vi "RLS_identificacion.vi"() -> ()   [LabVIEW 2022 SP3]
uses:
  <vilib>/Utility/NIReport.llb/Report Type.ctl
  <vilib>/imath/engines/lvmath2/RunTimeEngine/NodeEndStatement/NIMS_NodeEndStatement_Output.vi
  <instcachedir>/0/NIMS_NodeEndStatement_Output_53EC0D466D134D7ABD903AC30B43404B.lvgen/NIMS_NodeEndStatement_Output_53EC0D466D134D7ABD903AC30B43404B_001.vi
  <vilib>/imath/engines/lvmath2/RunTimeEngine/ErrorHandling/NIMS_Finalize Error.vi
  <vilib>/imath/engines/lvmath2/RunTimeEngine/Managers/WorkSpace/UID Generator.vi
  <vilib>/imath/engines/lvmath2/RunTimeEngine/RunTimeType/NIMS_RunTimeType_From StrictType (excl LVString).vi
  <instcachedir>/0/NIMS_RunTimeType_From StrictType (excl LVString)_70DEE8F51B6B495C85F505DE4E7061F1.lvgen/NIMS_RunTimeType_From StrictType (excl LVString)_70DEE8F51B6B495C85F505DE4E7061F1_000.vi
  <vilib>/imath/engines/lvmath2/RunTimeEngine/LocalVariableDefStatement/MC_LocalVariableDefStatement_Display.vi
  <vilib>/imath/engines/lvmath2/RunTimeEngine/ArithmeticOperatorToken/NIMS_ArithmeticOperator_multmx(RV,M).vi
  <instcachedir>/0/NIMS_ArithmeticOperator_multmx(RV,M)_0C5EC56C64A44F5D9A149E640905A95E.lvgen/NIMS_ArithmeticOperator_multmx(RV,M)_0C5EC56C64A44F5D9A149E640905A95E_001.vi
  <vilib>/imath/engines/lvmath2/RunTimeEngine/ArithmeticOperatorToken/NIMS_ArithmeticOperator_multmx(M,CV).vi
  <instcachedir>/0/NIMS_ArithmeticOperator_multmx(M,CV)_F5DBFFF0126A4383B39F7B34D5ABA6C8.lvgen/NIMS_ArithmeticOperator_multmx(M,CV)_F5DBFFF0126A4383B39F7B34D5ABA6C8_000.vi
  <vilib>/imath/engines/lvmath2/RunTimeEngine/ArithmeticOperatorToken/NIMS_ArithmeticOperator_rightdivmx.vi
  <instcachedir>/0/NIMS_ArithmeticOperator_rightdivmx_6089A681D87747958E3B9B6C89182D1F.lvgen/NIMS_ArithmeticOperator_rightdivmx_6089A681D87747958E3B9B6C89182D1F_000.vi
  <vilib>/imath/engines/lvmath2/RunTimeEngine/ErrorHandling/NIMS_Create Error From Enums.vi
  <vilib>/imathl/engines/lvmath/Functions/Error Handling/Create Error.vi
  <vilib>/imath/engines/lvmath2/RunTimeEngine/ArithmeticOperatorToken/NIMS_ArithmeticOperator_multmx.vi
  <instcachedir>/0/NIMS_ArithmeticOperator_multmx_BDE1B5075EB4429787EED704427CBD98.lvgen/NIMS_ArithmeticOperator_multmx_BDE1B5075EB4429787EED704427CBD98_004.vi
  <vilib>/imath/engines/lvmath2/RunTimeEngine/ArithmeticOperatorToken/NIMS_ArithmeticOperator_plus.vi
  <instcachedir>/0/NIMS_ArithmeticOperator_plus_3E2F46F6B6A2434E909AF418D4802C21.lvgen/NIMS_ArithmeticOperator_plus_3E2F46F6B6A2434E909AF418D4802C21_003.vi
  <vilib>/imath/engines/lvmath2/RunTimeEngine/ArithmeticOperatorToken/NIMS_ArithmeticOperator_minus.vi
  <instcachedir>/0/NIMS_ArithmeticOperator_minus_22EE3FD1C8824638A4ED1C446A3DB56D.lvgen/NIMS_ArithmeticOperator_minus_22EE3FD1C8824638A4ED1C446A3DB56D_009.vi
  <vilib>/imath/engines/lvmath2/RunTimeEngine/IndexRead/NIMS M(S).vi
  <instcachedir>/0/NIMS M(S)_B826C018497E4940AE96BD27B540B6FB.lvgen/NIMS M(S)_B826C018497E4940AE96BD27B540B6FB_000.vi
  <vilib>/imath/engines/lvmath2/RunTimeEngine/Managers/SymbolTable/Clear UID.vi
  <instcachedir>/0/NIMS_NodeEndStatement_Output_53EC0D466D134D7ABD903AC30B43404B.lvgen/NIMS_NodeEndStatement_Output_53EC0D466D134D7ABD903AC30B43404B_002.vi
  <vilib>/addons/_office/excel.llb/Excel Easy Table (num).vi
  <vilib>/Utility/NIReport.llb/NI_report.lvclass
  <vilib>/Utility/NIReport.llb/NI_ReportGenerationCore.lvlib
  <vilib>/Utility/NIReport.llb/Excel/NI_Excel.lvclass
  <vilib>/addons/_office/NI_ReportGenerationToolkit.lvlib
  <vilib>/imath/engines/lvmath2/RunTimeEngine/Managers/SymbolTable/NIMS_WorkSpace.lvlib
panel:
  in  "template (empty)":path
  in  "stop":bool
  in  "u(k)":dbl
  in  "Pertubación":bool
  in  "Tiempo de  ejecucion":u32
  out "ARX orden 2":cluster{"set-point ":dbl, dbl, dbl, dbl}(graph)
  out "tetak2":dbl[][](array[numeric])
  out "ARX orden 1":cluster{"set-point ":dbl, dbl, dbl, dbl}(graph)
  out "tetak":dbl[][](array[numeric])
  out "a11":dbl
  out "a1":dbl=-0.8261
  out "a2":dbl
  out "b1":dbl=0.008316
  out "b2":dbl=0.1498
  out "b11":dbl
  out "a12":dbl
  out "a22":dbl
  out "b12":dbl
  out "?":dbl
  # "Vector de parametros\nestimados"
  # "Vector de parametros\nestimados"
  # "Z+"
  # "Gp(Z) ="
  # "Gp(Z) ="
  # "Z +"
  # "Z^2 +"
  # "Z+"
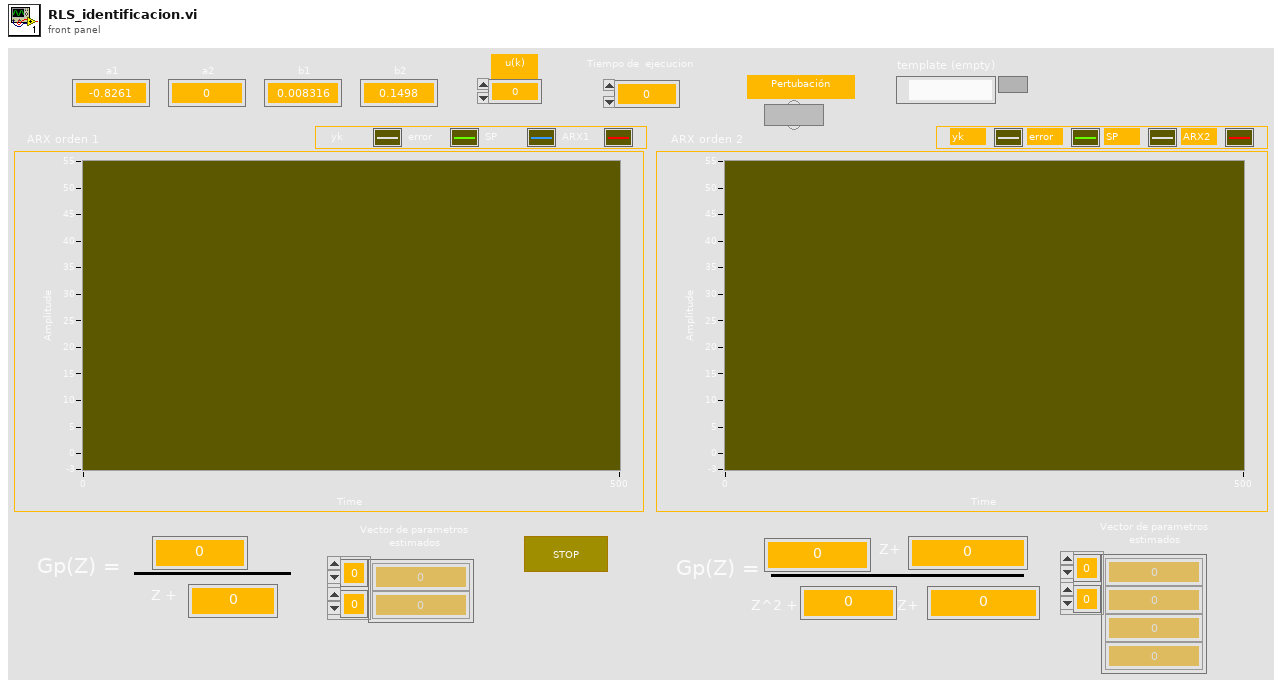
[diagram p1: front panel]
types:
  T1 = typedef "NI_ReportGenerationCore.lvlib/Report Type.ctl" = enum16{"HTML", "Word", "Excel"}
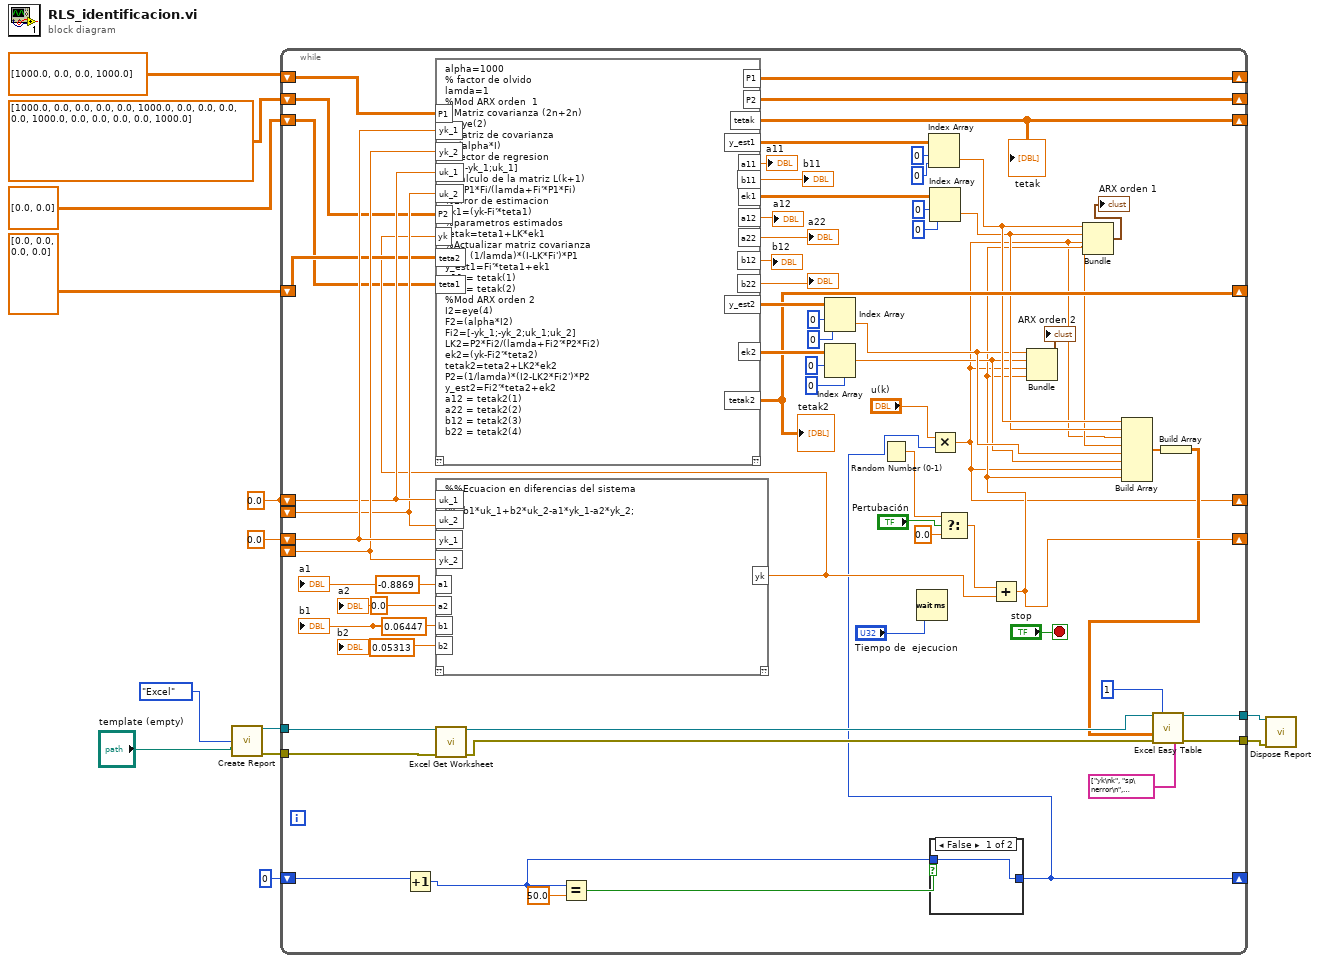
[diagram p0: block diagram]
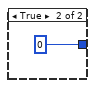
[diagram p2: hidden frame]
diagram:
  w9 = 0.0 ("set-point")
  w8 = 0.0 ("set-point")
  n1 = call <vilib>:"Create Report.vi"("report type"=Report_Type."Excel", "template (empty)"="template (empty)") -> ("report out"=w5:refnum<class "NI_report.lvclass">, "error out"=w4:errorcluster)  [unwired: 12 in]
  n2 = while {
    shift-right: [w29] -> _
    shift-left: w8 -> [w77]
    shift-left: w8 -> [w76]
    shift-right: [w19] -> _
    shift-left: w9 -> [w75]
    shift-left: w9 -> [w74]
    shift-right: [w59] -> _
    shift-left: dbl[][] [[0.0], [0.0], [0.0], [0.0]] ("tetak2") -> [w73]
    shift-right: [w58] -> _
    shift-left: dbl[][] [[1000.0, 0.0], [0.0, 1000.0]] ("P1") -> [w56]
    shift-right: [w57] -> _
    shift-left: dbl[][] [[1000.0, 0.0, 0.0, 0.0], [0.0, 1000.0, 0.0, 0.0], [0.0, 0.0, 1000.0, 0.0], [0.0, 0.0, 0.0, 1000.0]] ("P") -> [w55]
    shift-right: [w54] -> _
    shift-left: dbl[][] [[0.0], [0.0]] ("tetak") -> [w53]
    tunnel: w5 -> [w35]
    tunnel: w4 -> [w34]
    tunnel: [w22] -> w3
    tunnel: [w21] -> w2
    shift-right: [w14] -> _
    shift-left: 0 -> [w18]
    stop <- "stop" stop-if-true
    w41 = 0.05313 ("b2")
    w42 = 0.06447 ("b1")
    w43 = 0.0 ("a2")
    w44 = -0.8869 ("a1")
    n3 = Increment(x=w18) -> (x+1=w15:i32)
    n4 = mathscript code="%%Ecuacion en diferencias del sistema\n\nyk=b1*uk_1+b2*uk_2-a1*yk_1-a2*yk_2;"("uk_1"=w75, "uk_2"=w74, "yk_1"=w77, "yk_2"=w76, "a1"=w44, "a2"=w43, "b1"=w42, "b2"=w41) -> ("yk"=w62:dbl)  [unwired: 1 in, 1 out]
    n5 = mathscript code="alpha=1000\n% factor de olvido \nlamda=1\n%Mod ARX orden  1\n%Matriz covarianza (2n+2n)\nI=eye(2)\n%Matriz de covarianza \nF=(alpha*I)\n%Vector de regresion\nFi=[-yk_1;uk_1]\n%Calculo de la matriz L(k+1)\nLK=P1*Fi/(lamda+Fi'*P1*Fi)\n%Error de estimacion \nek1=(yk-Fi'*teta1)\n%parametros estimados \ntetak=teta1+LK*ek1\n%Actualizar matriz covarianza \nP1 = (1/lamda)*(I-LK*Fi')*P1\ny_est1=Fi'*teta1+ek1\na11 = tetak(1)\nb11 = tetak(2)\n%Mod ARX orden 2\nI2=eye(4)\nF2=(alpha*I2)\nFi2=[-yk_1;-yk_2;uk_1;uk_2]\nLK2=P2*Fi2/(lamda+Fi2'*P2*Fi2)\nek2=(yk-Fi2'*teta2)\ntetak2=teta2+LK2*ek2\nP2=(1/lamda)*(I2-LK2*Fi2')*P2\ny_est2=Fi2'*teta2+ek2\na12 = tetak2(1)\na22 = tetak2(2)\nb12 = tetak2(3)\nb22 = tetak2(4)"("yk_1"=w77, "yk_2"=w76, "uk_1"=w75, "uk_2"=w74, "P2"=w55, "yk"=w62, "teta2"=w73, "teta1"=w53, "P1"=w56) -> ("tetak2"=w59:dbl[][], "ek2"=w66:dbl[][], "y_est2"=w60:dbl[][], "P1"=w58:dbl[][], "P2"=w57:dbl[][], "tetak"=w54:dbl[][], "ek1"=w49:dbl[][], "y_est1"=w51:dbl[][], "a11"=→"a11":dbl, "b11"=→"b11":dbl, "a12"=→"a12":dbl, "a22"=→"a22":dbl, "b12"=→"b12":dbl, "b22"=→"?":dbl)  [unwired: 1 in, 1 out]
    "tetak2" <- w59
    "tetak" <- w54
    n6 = call <vilib>:"Excel Get Worksheet.vi"("report in"=w35, "error in (no error)"=w34) -> ("report out"=w25:refnum<class "NI_report.lvclass">, "error out"=w24:errorcluster)  [unwired: 12 in]
    n7 = Equal?(x=w15, y=50.0) -> (x = y?=w16:bool)
    n8 = Index Array(array=w60, index (row)=0 ("disabled index (row)"), index (col)=0 ("disabled index (col)")) -> (element=w31:dbl)
    n9 = Index Array(array=w66, index (row)=0, index (col)=0 ("disabled index (col)")) -> (element=w30:dbl)
    n10 = Random Number (0-1)() -> (number: 0 to 1=w67:dbl)
    n11 = Wait (ms)(milliseconds to wait="Tiempo de  ejecucion") -> ()  [unwired: 1 out]
    n12 = Index Array(array=w51, index (row)=0 ("disabled index (row)"), index (col)=0 ("disabled index (col)")) -> (element=w33:dbl)
    n13 = Index Array(array=w49, index (row)=0 ("disabled index (row)"), index (col)=0 ("disabled index (col)")) -> (element=w32:dbl)
    n14 = case shown="False" w16 {
      tunnel: [w79 0] -> w14
      tunnel: w15 -> [w79 _]
      frame False {
      }
      frame True {
      }
    }
    n15 = Multiply(x="u(k)", y=w14) -> (x*y=w19:dbl)
    n16 = Select(t=w67, s="Pertubación", f=0.0) -> (s? t:f=w68:dbl)
    n17 = Add(x=w68, y=w62) -> (x+y=w29:dbl)
    n18 = Bundle(w31, w30, w19, w29) -> (→"ARX orden 2":cluster{dbl, dbl, dbl, dbl})  [unwired: 1 in]
    n19 = Bundle(w33, w32, w19, w29) -> (→"ARX orden 1":cluster{dbl, dbl, dbl, dbl})  [unwired: 1 in]
    n20 = Build Array(w33, w32, w19, w29, w31, w30, w19, w29) -> (w28:dbl[])
    n21 = Build Array(w28) -> (w23:dbl[][])
    n22 = call-poly <vilib>:"Excel Easy Table.vi"("report in"=w25, "iteration"=1, "text data"=w23, "error in (no error)"=w24, "column headers"=string[] ["yk\nk", "sp\nerror\n", "errorsp\n", "ley cARX1\n", "YK2\n", "ERROR\n", "SP\n", "ARX2\n"]) -> ("report out"=w22:refnum<class "NI_report.lvclass">, "error out"=w21:errorcluster)  [unwired: 6 in, 3 out]
    "a1" <- w44
    "a2" <- w43
    "b1" <- w42
    "b2" <- w41
  }
  n23 = call-dynamic "Dispose Report.vi"("report in"=w3, "error in (no error)"=w2) -> ()  [unwired: 13 in, 1 out]
